vi "PromptUserPassFail.vi"   [LabVIEW 2015]
types:
  T1 = enum32{"Invalid", "Standard", "Closed", "Hidden", "Minimized", "Maximized"}
  T2 = enum32{"invalid app kind", "Development System", "Run Time System", "Student Edition", "Embedded LabVIEW", "Evaluation", "Custom"}
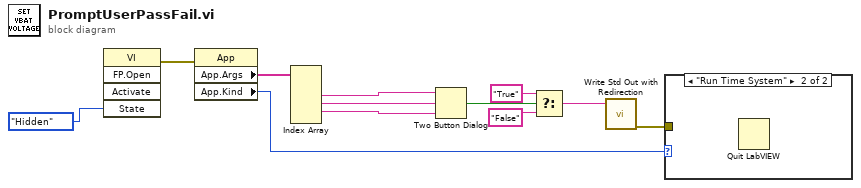
[diagram p0: block diagram]
diagram:
  n1 = invoke class="VI" method="FP.Open"("State"=T1."Hidden") -> (error out=w9:errorcluster)  [unwired: 4 in, 4 out]
  n2 = property class="App"(error in=w9) -> ("App.Args"=w12:string[], "App.Kind"=w11:T2)  [unwired: 1 in, 2 out]
  n3 = Index Array(array=w12) -> (element #2=w7:string, element #3=w6:string, element #4=w5:string)  [unwired: 5 in, 2 out]
  n4 = Two Button Dialog(message=w7, 1:w5, 2:w6) -> (T button?=w4:bool)
  n5 = Select(t="True", s=w4, f="False") -> (s? t:f=w1:string)
  n6 = call "Write Std Out with Redirection.vi"("string"=w1) -> ("error out"=w10:errorcluster)  [unwired: 10 in]
  n7 = case shown="\"Run Time System\"" w11 {
    tunnel: w10 -> [_ _]
    frame Default {
    }
    frame "Run Time System" {
      n8 = Quit LabVIEW() -> ()  [unwired: 1 in]
    }
  }
